vi "LSX Get Status TVRO.vi"(8 "error in (no error)":errorcluster, 9 "lMaxLen":i32, 10 "pcStat":string, 11 "lLSID":i32) -> (0 "error out":errorcluster, 2 "pcStat out":string, 3 "function return":i32)   [LabVIEW 2018, in "Tango.lvlib"]
doc: "TANGOAPI int TANGOCALL LSX_GetStatusTVRO (int lLSID, char *pcStat, int lMaxLen);"
uses:
  <userlib>/Tango/Tango.lvlib
  <userlib>/Tango/Tango_DLL.dll
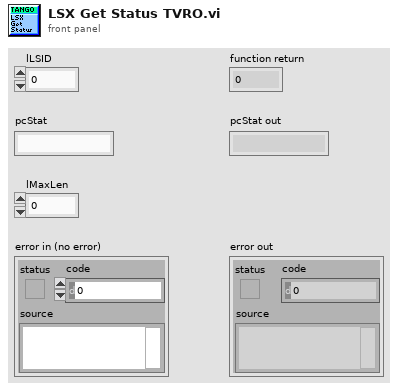
[diagram p1: front panel]
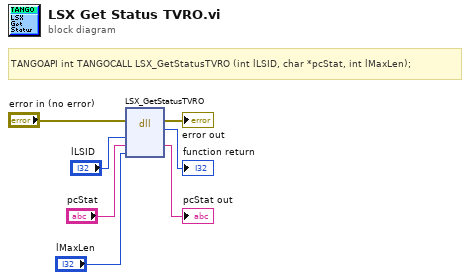
[diagram p0: block diagram]
diagram:
  # "TANGOAPI int TANGOCALL LSX_GetStatusTVRO (int lLSID, char *pcStat, int lMaxLen);"
  n1 = dll-call lib="C:/Program Files (x86)/National Instruments/LabVIEW 2018/user.lib/Tango/Tango_DLL.*" fn="LSX_GetStatusTVRO"(error in="error in (no error)", "lLSID"="lLSID", "pcStat"="pcStat", "lMaxLen"="lMaxLen") -> (error out=→"error out":errorcluster, →"function return":i32, "pcStat"=→"pcStat out":string)  [unwired: 4 in, 1 out]
